vi "Update Elapsed Time.vi"(8 "error in (no error)":errorcluster, 10 "Elapsed Time":dbl, 11 "Chef Actor in":refnum<class "Chef Actor.lvclass">) -> (0 "error out":errorcluster, 3 "Chef Actor out":refnum<class "Chef Actor.lvclass">)   [LabVIEW 2024, in "Chef Actor.lvlib" / "Chef Actor.lvclass"]
uses:
  Chef Actor.lvclass
  Chef Actor.lvclass/Chef Actor.ctl
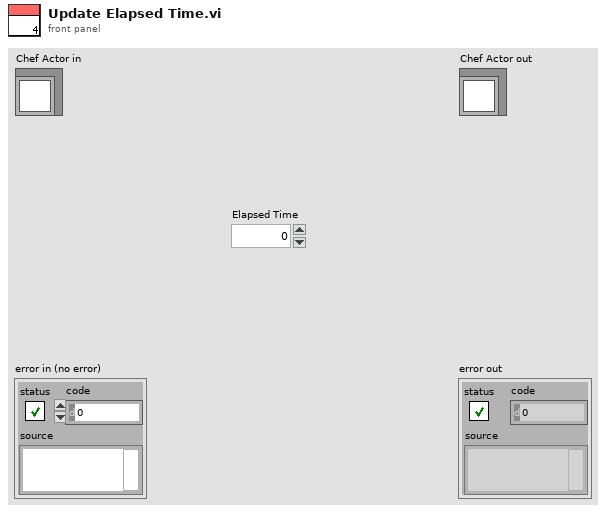
[diagram p1: front panel]
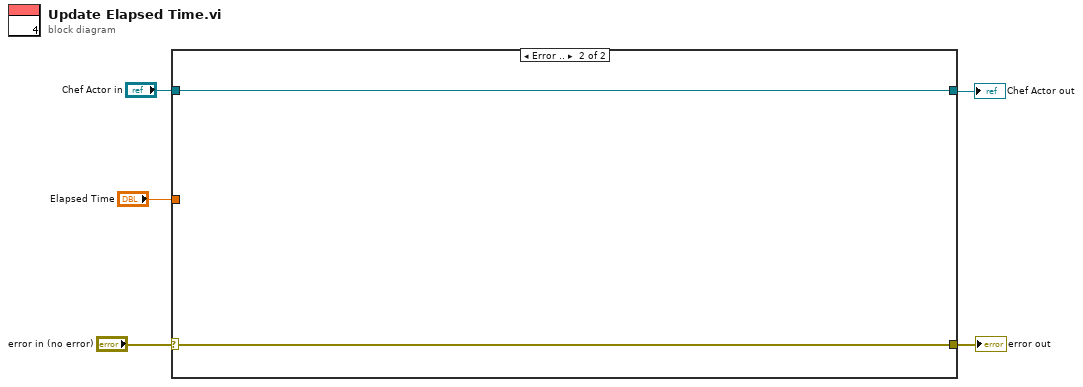
[diagram p0: block diagram]
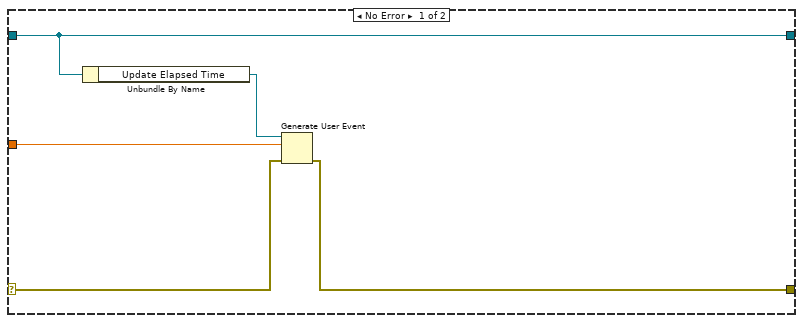
[diagram p2: hidden frame]
diagram:
  n1 = case shown="Error .." "error in (no error)" {
    selector: "error in (no error)" -> [w7 w11]
    tunnel: [w10 w12] -> w3
    tunnel: "Chef Actor in" -> [w10 w12]
    tunnel: "Elapsed Time" -> [w8 _]
    tunnel: [w6 w11] -> w1
    frame No Error {
      n2 = Unbundle By Name(w10) -> ("Update Elapsed Time"=w9:refnum<user-event>)
      n3 = Generate User Event(user event=w9, event data cluster=w8, error in=w7) -> (error out=w6:errorcluster)  [unwired: 1 in, 1 out]
    }
    frame Error {
    }
  }
  "error out" <- w1
  "Chef Actor out" <- w3
